vi "initSingle.vi"(8 "errorIn":errorcluster, 10 "name":string="name", 11 "size(-1)":i32) -> (0 "errorOut":errorcluster, 3 "refer":refnum<queue>)   [LabVIEW 2017]
uses:
  models/EMSGData.ctl
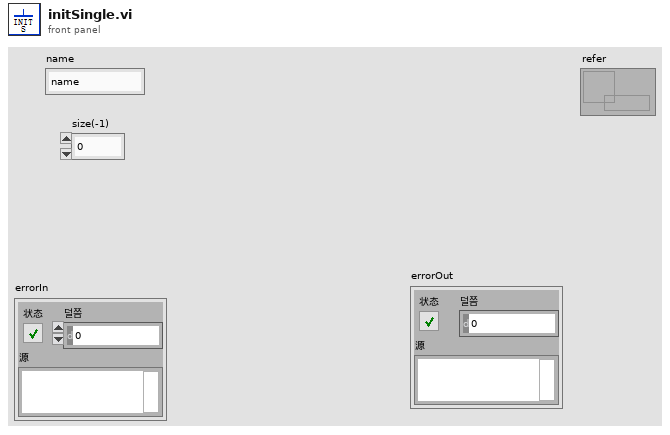
[diagram p1: front panel]
types:
  T1 = typedef "EMSGData.ctl" = cluster{"to":string, "from":string, "data":variant, "remark1":string, "remark 2":string}
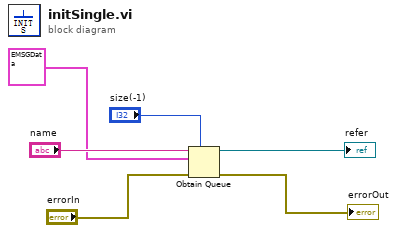
[diagram p0: block diagram]
diagram:
  n1 = Obtain Queue(max queue size (-1, unlimited)="size(-1)", name (unnamed)="name", element data type=T1 {"to"="", "from"="", "data"=variant, "remark1"="", "remark 2"=""} ("EMSGData"), error in (no error)="errorIn") -> (queue out=→"refer":refnum<queue>, error out=→"errorOut":errorcluster)  [unwired: 1 in, 1 out]
